vi "close panels.vi"(8 "error in":errorcluster, 11 "vi refs":refnum<vi>[](array[refnum])) -> (0 "error out":errorcluster)   [LabVIEW 2017]
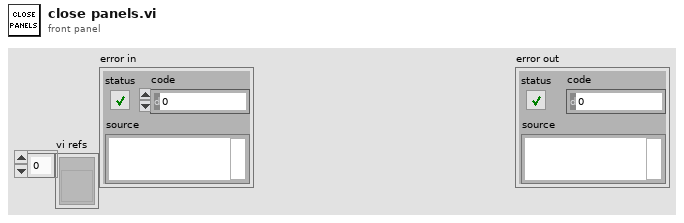
[diagram p1: front panel]
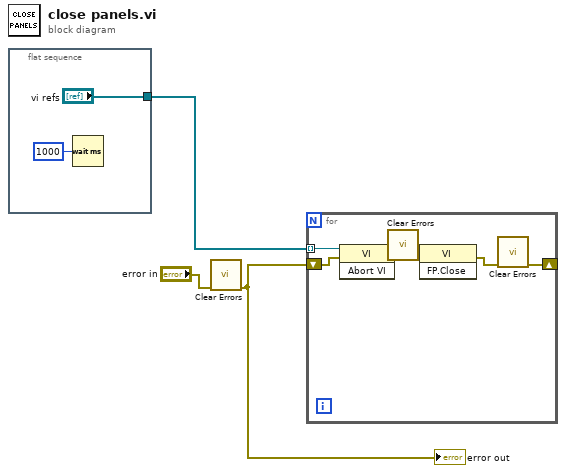
[diagram p0: block diagram]
diagram:
  n1 = flat-sequence {
    tunnel: ["vi refs"] -> w3
    frame #0 {
      n2 = Wait (ms)(milliseconds to wait=u32 1000) -> ()  [unwired: 1 out]
    }
  }
  n3 = call <vilib>:"Clear Errors.vi"("error in (no error)"="error in") -> ("error out"=w1:errorcluster)  [unwired: 5 in, 1 out]
  "error out" <- w1
  n4 = for {
    tunnel: w3 -> [w12] mode=indexing
    shift-right: [w8] -> _
    shift-left: w1 -> [w7]
    n5 = invoke class="VI" method="Abort VI"(reference=w12, error in=w7) -> (reference out=w11:refnum<vi>, error out=w10:errorcluster)  [unwired: 1 in, 1 out]
    n6 = call <vilib>:"Clear Errors.vi"("error in (no error)"=w10) -> ("error out"=w6:errorcluster)  [unwired: 5 in, 1 out]
    n7 = invoke class="VI" method="FP.Close"(reference=w11, error in=w6) -> (error out=w9:errorcluster)  [unwired: 1 in, 2 out]
    n8 = call <vilib>:"Clear Errors.vi"("error in (no error)"=w9) -> ("error out"=w8:errorcluster)  [unwired: 5 in, 1 out]
  }
